vi "Set Up Dialog - Polar Heart Rate.vi"() -> ()   [LabVIEW 2012]
panel:
  out "Calibration Instructions":string="1. Connect the sensor to your myDAQ as shown in the diagram above. Plug the 1/8 in audio connector (headphone jack) into the adaptor cable then plug the cable into the iWorx Sensor Adaptor.\n\n2. Wrap the heart monitor band around your chest so that it touches your bare skin around the sternum. Make sure the sensor is snapped onto the band.\n\n3. Wait for the signal to appear then press the Calibrate button to automatically set the threshold limit. You should see a large negative spike with each heartbeat."
  # "iWorx - Polar Hear Rate Monitor - Set Up"
  # "Polar Hear Rate Monitor (PHRMN - 100)"
  # "iWorx"
  # "Sensor"
  # "PHRMN - 100"
  # "myDAQ"
  # "Computer"
  # "Adaptor"
  # "Connection Diagram"
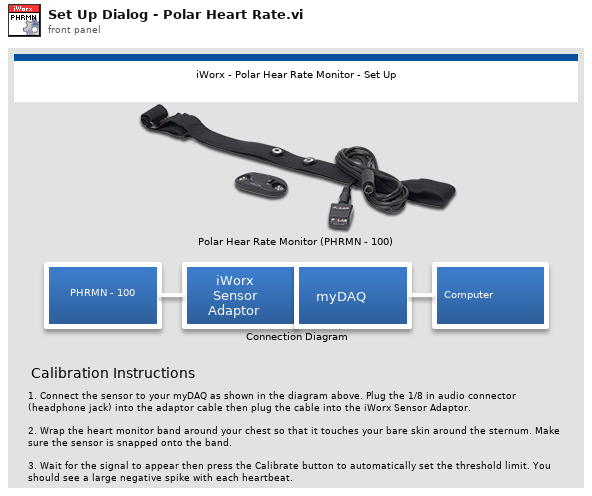
[diagram p1: front panel]
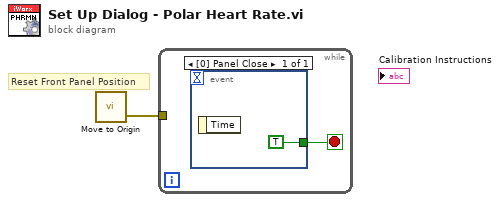
[diagram p0: block diagram]
diagram:
  # "Reset Front Panel Position"
  n1 = call "Move to Origin.vi"() -> ("Error Out"=w1:errorcluster)  [unwired: 3 in]
  n2 = while {
    tunnel: w1 -> [_]
    stop <- w2 stop-if-true
    n3 = event shown="[0] Panel Close" {
      selector: _ -> [_]
      dyn-events: _ -> [_]
      timeout: _ -> [_]
      tunnel: [TRUE] -> w2
      event Panel Close {
        n4 = event-data() -> ()  [unwired: 1 in, 1 out]
      }
    }
  }
